vi "gantry_home.vi"(7 "lines":tag, 8 "VISA resource name 2":refnum<visa-resource-name>, 10 "dir":dbl=1.0, 11 "desired motor speed (T/2) [us]":dbl=250.0) -> (0 "VISA resource name":refnum<visa-resource-name>)   [LabVIEW 2021]
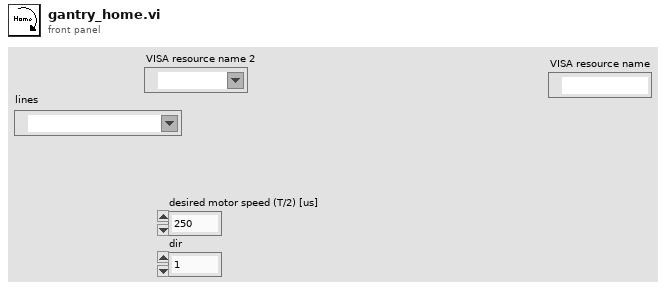
[diagram p1: front panel]
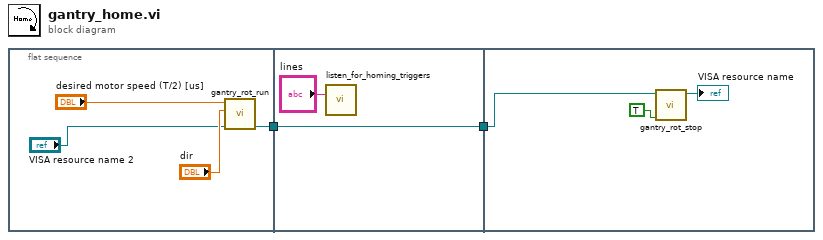
[diagram p0: block diagram]
diagram:
  n1 = flat-sequence {
    tunnel: [w3] -> w1
    tunnel: [w8] -> w2
    tunnel: w1 -> [w8]
    tunnel: w2 -> [w9]
    frame #0 {
      n2 = call "gantry_rot_run.vi"("VISA resource name"="VISA resource name 2", "dir"="dir", "desired motor speed (T/2) [us]"="desired motor speed (T/2) [us]") -> ("VISA resource name out"=w3:refnum<visa-resource-name>)  [unwired: 7 in, 1 out]
    }
    frame #1 {
      n3 = call "listen_for_homing_triggers.vi"("lines"="lines") -> ()  [unwired: 11 in]
    }
    frame #2 {
      n4 = call "gantry_rot_stop.vi"("Rapid stop?"=TRUE, "VISA resource name"=w9) -> ("VISA resource name out"=→"VISA resource name":refnum<visa-resource-name>)  [unwired: 9 in]
    }
  }
